vi "Fit VI window to Largest Dec.vi"(4 "error in (no error)":errorcluster, 6 "border spacing (2 px)":i32=2, 7 "VI Ref (calling VI)":refnum<vi>) -> (0 "error out":errorcluster, 3 "VI Ref out":refnum<vi>)   [LabVIEW 2017]
doc: "Resizes and centres the VI window around the largest decoration on the front panel, adding the configured border spacing in pixels. It is a no-op when no decoration is found, and it cannot see locked decorations."
panel:
  # "Fit VI window to Largest Decoration.vi\n\nFits a VI's front panel window to its largest decoration size.\n\nPlease visit http://www.OpenG.org to learn about the\nOpen Source LabVIEW software movement.\n\nNOTICE -- YOU MUST LEAVE THIS NOTICE IN PLACE.  PER THE TERMS OF THE LICENSE BELOW, YOU MAY SUBLICENSE THIS SOFTWARE \nIN ANY WAY THAT DOES NOT CONFLICT WITH THIS LICENSE.\n\n### BSD License (http://www.opensource.org/licenses/bsd-license.php) Begin ###\n \nCopyright (c) 2002, Jim Kring <jim@jimkring.com>\nCopyright (c) 2002, Cal-Bay Systems, Inc. <info@calbay.com>\n\nAll rights reserved.\n\nRedistribution and use in source and binary forms, with or without modification, are permitted provided that the following conditions are met:\n\n    * Redistributions of source code must retain the above copyright notice, this list of conditions and the following disclaimer.\n    * Redistributions in binary form must reproduce the above copyright notice, this list of conditions and the following disclaimer in the \n       documentation and/or other materials provided with the distribution.\n    * Neither the name of SciWare, James Kring, Inc., nor the names of its contributors may be used to endorse or promote products derived \n       from this software without specific prior written permission.\n\nTHIS SOFTWARE IS PROVIDED BY THE COPYRIGHT HOLDERS AND CONTRIBUTORS \"AS IS\" AND ANY EXPRESS OR IMPLIED WARRANTIES, \nINCLUDING, BUT NOT LIMITED TO, THE IMPLIED WARRANTIES OF MERCHANTABILITY AND FITNESS FOR A PARTICULAR PURPOSE ARE \nDISCLAIMED. IN NO EVENT SHALL THE COPYRIGHT OWNER OR CONTRIBUTORS BE LIABLE FOR ANY DIRECT, INDIRECT, INCIDENTAL,\n SPECIAL, EXEMPLARY, OR CONSEQUENTIAL DAMAGES (INCLUDING, BUT NOT LIMITED TO, PROCUREMENT OF SUBSTITUTE GOODS OR \nSERVICES; LOSS OF USE, DATA, OR PROFITS; OR BUSINESS INTERRUPTION) HOWEVER CAUSED AND ON ANY THEORY OF LIABILITY, \nWHETHER IN CONTRACT, STRICT LIABILITY, OR TORT (INCLUDING NEGLIGENCE OR OTHERWISE) ARISING IN ANY WAY OUT OF THE USE \nOF THIS SOFTWARE, EVEN IF ADVISED OF THE POSSIBILITY OF SUCH DAMAGE.\n\n### BSD License End ###"
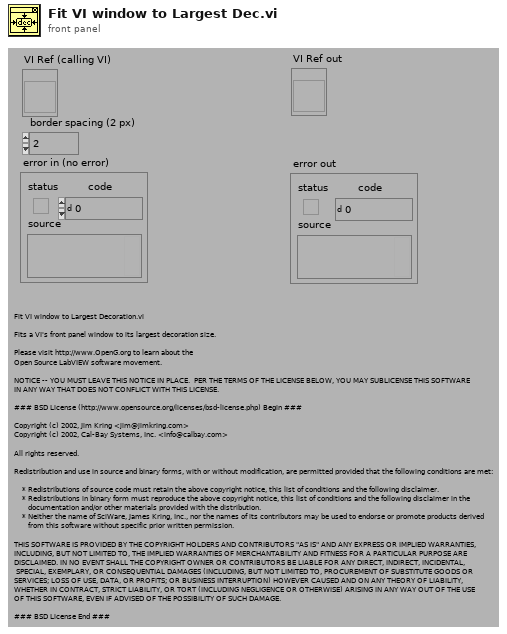
[diagram p1: front panel]
types:
  T1 = typedef "LVRectTypeDef.ctl" = cluster{"Left":i16, "Top":i16, "Right":i16, "Bottom":i16}
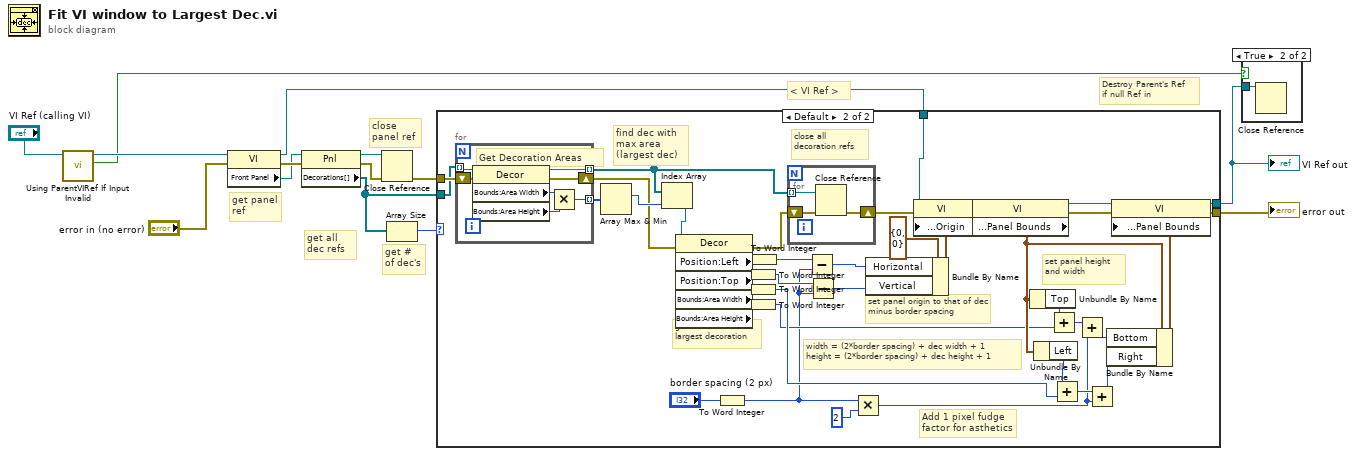
[diagram p0: block diagram]
diagram:
  # "Destroy Parent's Ref\nif null Ref in"
  # "get # of dec's"
  # "get panel ref"
  # "get all dec refs"
  # "close panel ref"
  # "< VI Ref >"
  n1 = call "Using ParentVIRef If Input Invalid.vi"("VI Ref (calling VI)"="VI Ref (calling VI)") -> ("Using Parent Ref(Need to Destroy)"=w1:bool, "VI Ref"=w2:refnum<vi>)  [unwired: 5 in]
  n2 = property on="Property Node" class="VI"(reference=w2, error in="error in (no error)") -> (reference out=w14:refnum<vi>, error out=w12:errorcluster, "Front Panel"=w9:refnum<vi>)
  n3 = property on="Property Node" class="Pnl"(reference=w9, error in=w12) -> (reference out=w13:refnum<vi>, error out=w11:errorcluster, "Decorations[]"=w6:refnum<vi>[])
  n4 = Close Reference(reference=w13, error in (no error)=w11) -> (error out=w8:errorcluster)
  n5 = Array Size(array=w6) -> (size(s)=w5:i32)
  n6 = case shown="Default" w5 {
    tunnel: w14 -> [w16 w54]
    tunnel: w8 -> [w15 w37]
    tunnel: [w15 w25] -> w7
    tunnel: [w16 w24] -> w3
    tunnel: w6 -> [_ w23]
    frame 0 {
      # "do nothing if no decorations"
    }
    frame Default {
      # "width = (2*border spacing) + dec width + 1\nheight = (2*border spacing) + dec height + 1"
      # "set panel height and width"
      # "set panel origin to that of dec minus border spacing"
      # "close all  decoration refs"
      # "get coord's of largest decoration"
      # "Add 1 pixel fudge factor for asthetics"
      # "find dec with max area (largest dec)"
      n7 = for {
        tunnel: w23 -> [w63] mode=indexing
        tunnel: [w60] -> w36 mode=indexing
        shift-right: [w58] -> w32
        shift-left: w37 -> [w59]
        tunnel: [w57] -> w34 mode=indexing
        # "Get Decoration Areas"
        n8 = property class="Decor"(reference=w63, error in=w59) -> (reference out=w57:refnum<vi>, error out=w58:errorcluster, "Bounds:Area Width"=w62:u32, "Bounds:Area Height"=w61:u32)
        n9 = Multiply(x=w62, y=w61) -> (x*y=w60:u32)
      }
      n10 = Array Max & Min(array=w36) -> (max index (indices)=w35:i32)  [unwired: 3 out]
      n11 = Index Array(array=w34, index=w35) -> (element=w33:refnum<vi>)
      n12 = property class="Decor"(reference=w33, error in=w32) -> (error out=w31:errorcluster, "Position:Left"=w40:i32, "Position:Top"=w43:i32, "Bounds:Area Width"=w48:u32, "Bounds:Area Height"=w46:u32)  [unwired: 1 out]
      n13 = To Word Integer(number="border spacing (2 px)") -> (16bit integer=w17:i16)
      n14 = To Word Integer(number=w43) -> (16bit integer=w18:i16)
      n15 = To Word Integer(number=w48) -> (16bit integer=w21:i16)
      n16 = To Word Integer(number=w46) -> (16bit integer=w20:i16)
      n17 = To Word Integer(number=w40) -> (16bit integer=w19:i16)
      n18 = for {
        tunnel: w34 -> [w66] mode=indexing
        shift-right: [w64] -> w28
        shift-left: w31 -> [w65]
        n19 = Close Reference(reference=w66, error in (no error)=w65) -> (error out=w64:errorcluster)
      }
      n20 = Subtract(x=w19, y=w17) -> (x-y=w41:i16)
      n21 = Subtract(x=w18, y=w17) -> (x-y=w42:i16)
      n22 = Multiply(x=w17, y=i16 2) -> (x*y=w22:i16)
      n23 = Bundle By Name(cluster=cluster{"Horizontal":i16, "Vertical":i16} {"Horizontal"=0, "Vertical"=0} ("Front Panel Window:Origin"), "Horizontal"=w41, "Vertical"=w42) -> (w38:cluster{"Horizontal":i16, "Vertical":i16})
      n24 = property on="Property Node" class="VI"(reference=w54, error in=w28, "Front Panel Window:Origin"=w38) -> (reference out=w55:refnum<vi>, error out=w27:errorcluster)
      n25 = property on="Property Node" class="VI"(reference=w55, error in=w27) -> (reference out=w56:refnum<vi>, error out=w26:errorcluster, "Front Panel Window:Panel Bounds"=w44:T1)
      n26 = Unbundle By Name(w44) -> ("Top"=w45:i16)
      n27 = Unbundle By Name(w44) -> ("Left"=w47:i16)
      n28 = Add(x=w45, y=w20) -> (x+y=w52:i16)
      n29 = Add(x=w47, y=w21) -> (x+y=w50:i16)
      n30 = Add(x=w52, y=w22) -> (x+y=w53:i16)
      n31 = Add(x=w50, y=w22) -> (x+y=w51:i16)
      n32 = Bundle By Name(cluster=w44, "Bottom"=w53, "Right"=w51) -> (w49:T1)
      n33 = property on="Property Node" class="VI"(reference=w56, error in=w26, "Front Panel Window:Panel Bounds"=w49) -> (reference out=w24:refnum<vi>, error out=w25:errorcluster)
    }
  }
  "error out" <- w7
  "VI Ref out" <- w3
  n34 = case shown="True" w1 {
    tunnel: w3 -> [_ w67]
    frame False {
    }
    frame True {
      n35 = Close Reference(reference=w67) -> ()  [unwired: 1 in, 1 out]
    }
  }
